vi "BK Precision 8600 Series Monitor Input.vi"() -> ()   [LabVIEW 2018]
doc: "Exemplifies monitoring the input voltage and current in constant current mode."
uses:
  <instrlib>/BK Precision 8600 Series/BK Precision 8600 Series.lvlib
panel:
  in  "CC Current (0)":dbl min=0.0 max=720.0 step=1.0 format="%#.3f"
  out "Current":dbl
  out "Voltage":dbl format="%_6f"
  in  "?":bool
  in  "VISA resource name":refnum<visa-resource-name>
  in  "Serial Configuration":cluster{"Baud Rate":u32}={"Baud Rate"=9600} {"Baud Rate" items=["300"=300, "600"=600, "1200"=1200, "2400"=2400, "4800"=4800, "9600"=9600, "19200"=19200]}
  # "(c) 2014-2019 B&K Precision Corporation.  ALL RIGHTS RESERVED."
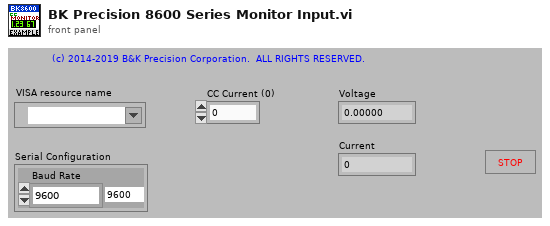
[diagram p1: front panel]
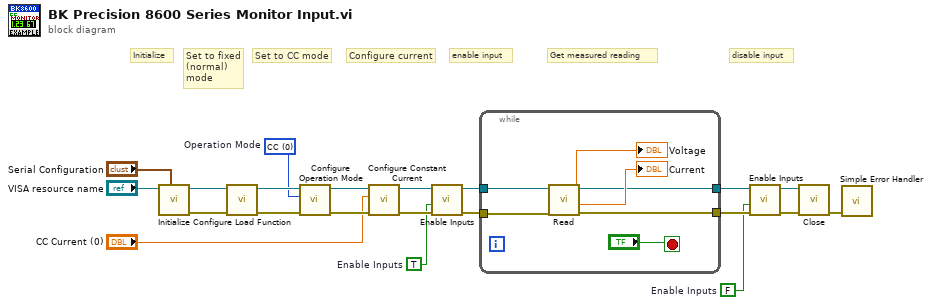
[diagram p0: block diagram]
diagram:
  w2 = u16 0 items=["CC", "CV", "CR", "CW", "CZ"]  # Operation Mode
  w3 = TRUE  # Enable Inputs
  w4 = FALSE  # Enable Inputs
  # "disable input"
  # "Get measured reading"
  # "enable input"
  # "Configure current"
  # "Set to CC mode"
  # "Set to fixed\n(normal)\nmode"
  # "Initialize"
  n1 = call <instrlib>:"Initialize.vi"("Serial Configuration"="Serial Configuration", "VISA resource name"="VISA resource name") -> ("error out"=w18:errorcluster, "VISA resource name out"=w19:refnum<visa-resource-name>)  [unwired: 8 in]
  n2 = call <instrlib>:"Configure Load Function.vi"("error in (no error)"=w18, "VISA resource name"=w19) -> ("error out"=w16:errorcluster, "VISA resource name out"=w17:refnum<visa-resource-name>)  [unwired: 8 in]
  n3 = call <instrlib>:"Configure Operation Mode.vi"("error in (no error)"=w16, "Operation Mode (0:CC)"=w2, "VISA resource name"=w17) -> ("error out"=w11:errorcluster, "VISA resource name out"=w12:refnum<visa-resource-name>)  [unwired: 7 in]
  n4 = call <instrlib>:"Configure Constant Current.vi"("error in (no error)"=w11, "CC Current (0)"="CC Current (0)", "VISA resource name"=w12) -> ("error out"=w9:errorcluster, "VISA resource name out"=w10:refnum<visa-resource-name>)  [unwired: 7 in]
  n5 = call <instrlib>:"Enable Inputs.vi"("error in (no error)"=w9, "Enable Input (F: False)"=w3, "VISA resource name"=w10) -> ("error out"=w7:errorcluster, "VISA resource name out"=w8:refnum<visa-resource-name>)  [unwired: 7 in]
  n6 = while {
    tunnel: w8 -> [w26]
    tunnel: w7 -> [w25]
    tunnel: [w24] -> w5
    tunnel: [w23] -> w6
    stop <- "?" stop-if-true
    n7 = call <instrlib>:"Read.vi"("error in (no error)"=w25, "VISA resource name"=w26) -> ("error out"=w24:errorcluster, "Current"=→"Current":dbl, "Voltage"=→"Voltage":dbl, "VISA resource name out"=w23:refnum<visa-resource-name>)  [unwired: 6 in]
  }
  n8 = call <instrlib>:"Enable Inputs.vi"("error in (no error)"=w5, "Enable Input (F: False)"=w4, "VISA resource name"=w6) -> ("error out"=w14:errorcluster, "VISA resource name out"=w13:refnum<visa-resource-name>)  [unwired: 7 in]
  n9 = call <instrlib>:"Close.vi"("error in (no error)"=w14, "VISA resource name"=w13) -> ("error out"=w15:errorcluster)  [unwired: 9 in]
  n10 = call <vilib>:"Simple Error Handler.vi"("error in (no error)"=w15) -> ()  [unwired: 4 in, 5 out]
